vi "axis to can.vi"(5 "send speed over can":T1, 6 "ROS":bool, 7 "wej auto":T2 {"zadany" format="%<%H:%M:%S\n%x>T"}, 8 "wej ster":cluster{"Y axis":dbl, "X axis":dbl}, 9 "wej  ID":T5, 10 "wej wagi":T4, 11 "ROS in":cluster{dbl, dbl}) -> (0 "array of cans":T6[](array[typedef]) {"type" items=["CAN Data", "CAN Remote"]; "identifier" format="%.0x"}, 2 "wyj pred":cluster{i16, i16, i16, i16, i16, i16} {"?" scale=-32767.0..32767.0; "?" scale=-32767.0..32767.0; "?" scale=-32767.0..32767.0; "?" scale=-32767.0..32767.0; "?" scale=-32767.0..32767.0; "?" scale=-32767.0..32767.0}, 3 "wyj auto":T3, 4 "wyœlij":bool=TRUE)   [LabVIEW 2015]
uses:
  CANFrameControl.ctl
  PC/wyj auto.ctl
panel:
  in  "reset":bool
  out "Time has Elapsed":bool
  out "Elapsed Time (s)":dbl
  out "zadany czas":bool
  out "AUTO ?":bool
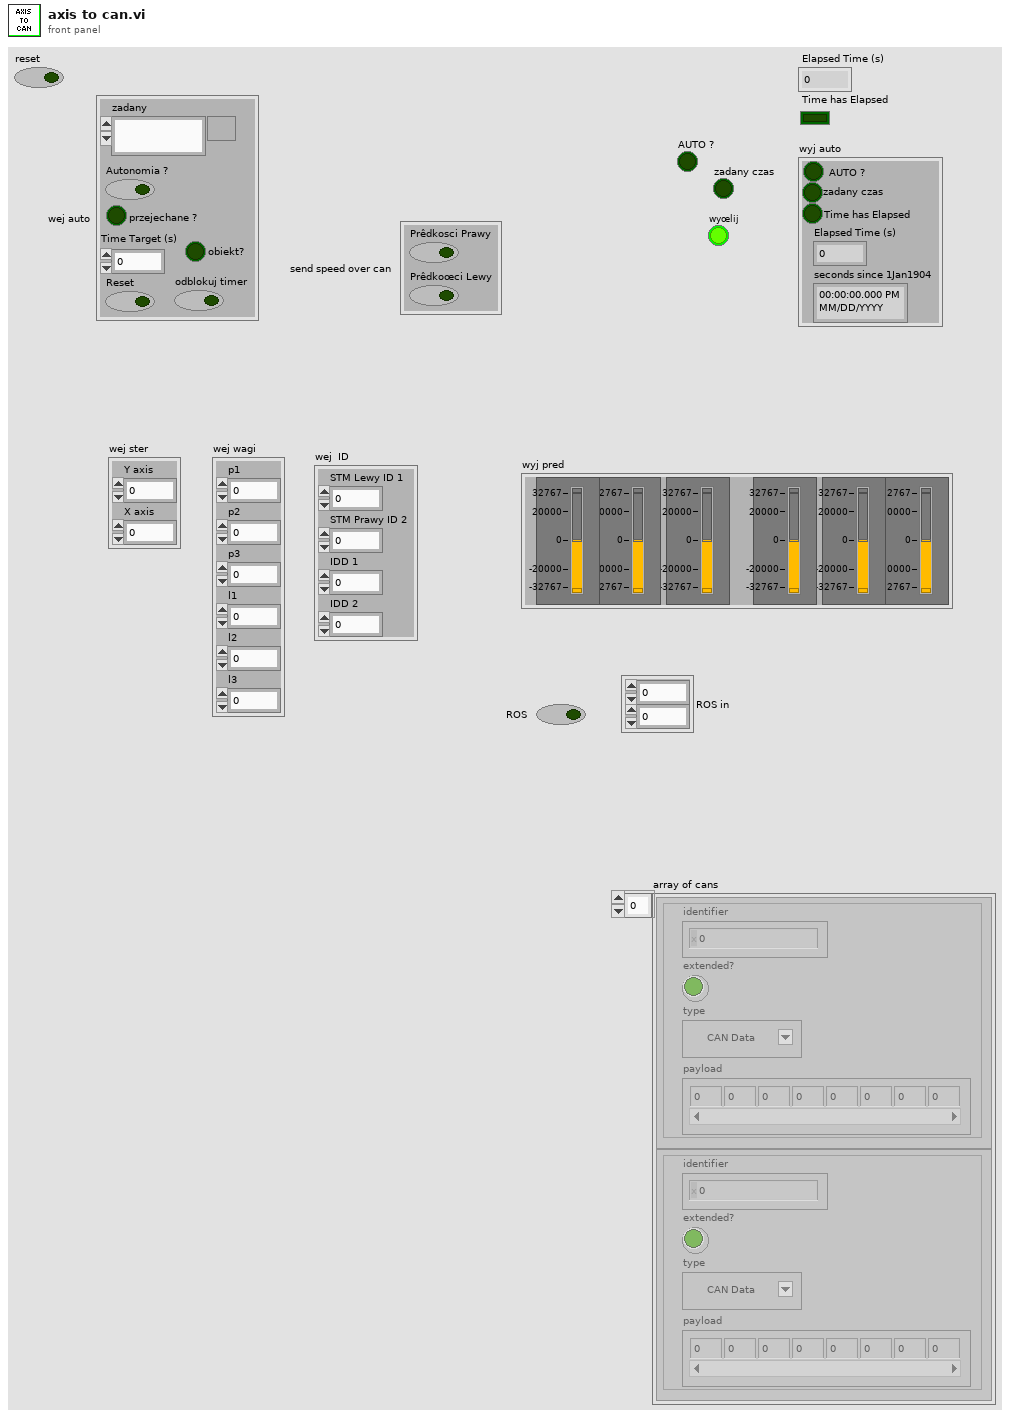
[diagram p1: front panel]
types:
  T1 = cluster{"Prêdkosci Prawy":bool, "Prêdkoœci Lewy":bool}
  T2 = cluster{"zadany":timestamp, "Autonomia ?":bool, "Time Target (s)":dbl, "Reset":bool, "odblokuj timer":bool, "obiekt?":bool, "przejechane ? ":bool}
  T3 = typedef "wyj auto.ctl" = cluster{"AUTO ?":bool, "zadany czas":bool, "Time has Elapsed":bool, "Elapsed Time (s)":dbl, "seconds since 1Jan1904":timestamp}
  T4 = cluster{"p1":dbl, "p2":dbl, "p3":dbl, "l1":dbl, "l2":dbl, "l3":dbl}
  T5 = cluster{"STM Lewy ID 1":u32, "STM Prawy ID 2":u32, "IDD 1":u8, "IDD 2":u8}
  T6 = typedef "CANFrameControl.ctl" = cluster{"identifier":u32, "extended?":bool, "type":u8, "payload":u8[]}
  T7 = cluster{bool, bool, "Time has Elapsed":bool, "Elapsed Time (s)":dbl, "seconds since 1Jan1904":timestamp}
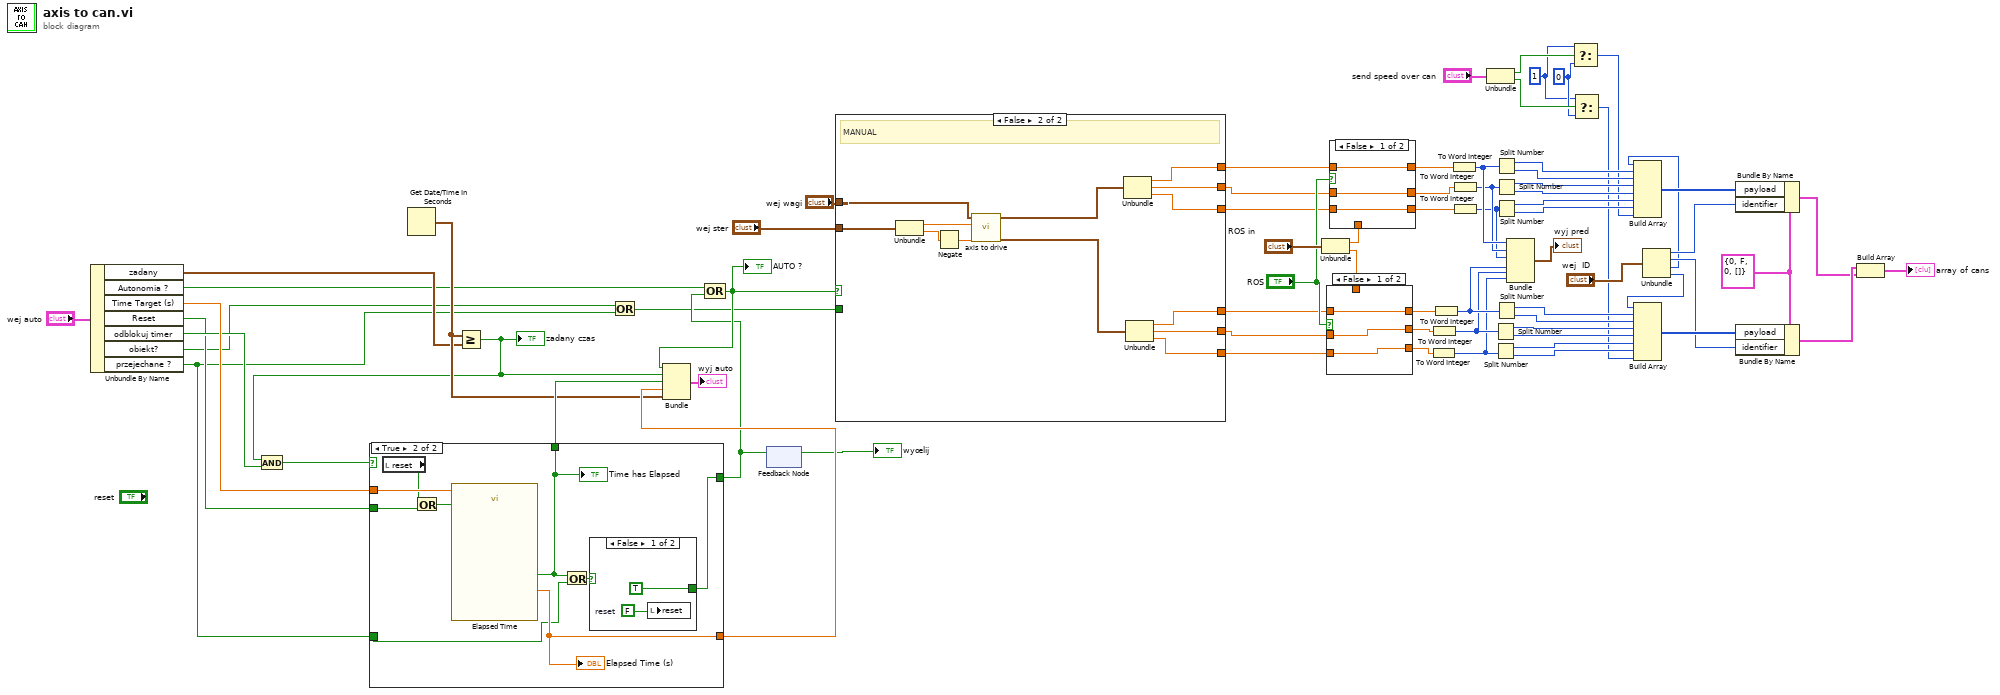
[diagram p0: block diagram]
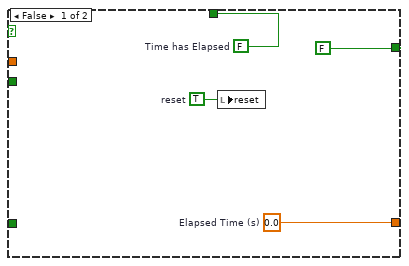
[diagram p4: hidden frame]
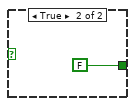
[diagram p5: hidden frame]
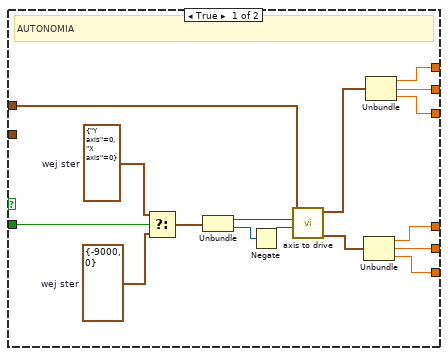
[diagram p6: hidden frame]
diagram:
  w17 = u8 1 ("element")
  w18 = u8 0 ("element")
  w72 = T6 {"identifier"=0, "extended?"=FALSE, "type"=0, "payload"=[]} ("CAN frame 2")
  n1 = Unbundle By Name("wej auto") -> ("zadany"=w36:timestamp, "Autonomia ?"=w31:bool, "Time Target (s)"=w38:dbl, "Reset"=w29:bool, "odblokuj timer"=w33:bool, "obiekt?"=w26:bool, "przejechane ?"=w24:bool)
  n2 = Get Date/Time In Seconds() -> (seconds since 1Jan1904=w37:timestamp)
  n3 = Greater Or Equal?(x=w37, y=w36) -> (x >= y?=w34:bool)
  "zadany czas" <- w34
  n4 = And(x=w34, y=w33) -> (x .and. y?=w35:bool)
  n5 = case shown="True" w35 {
    tunnel: [FALSE w86] -> w30
    tunnel: [w75 w80] -> w41
    tunnel: [w76 w79] -> w40
    tunnel: w29 -> [_ w83]
    tunnel: w38 -> [_ w85]
    tunnel: w24 -> [_ w78]
    frame False {
      w74 = TRUE  # reset
      w76 = 0.0  # Elapsed Time (s)
      w75 = FALSE  # Time has Elapsed
      n6 = local write "reset"(w74) -> ()
    }
    frame True {
      n7 = local read "reset"() -> (w82:bool)
      n8 = Or(x=w82, y=w83) -> (x .or. y?=w84:bool)
      n9 = call "Elapsed Time"("Time Target (s)"=w85, "Reset"=w84) -> ("Elapsed Time (s)"=w79:dbl, "Time has Elapsed"=w80:bool)  [unwired: 10 in, 6 out]
      "Elapsed Time (s)" <- w79
      "Time has Elapsed" <- w80
      n10 = Or(x=w80, y=w78) -> (x .or. y?=w81:bool)
      n11 = case shown="False" w81 {
        tunnel: [TRUE FALSE] -> w86
        frame False {
          w87 = FALSE  # reset
          n12 = local write "reset"(w87) -> ()
        }
        frame True {
        }
      }
    }
  }
  n13 = Or(x=w26, y=w24) -> (x .or. y?=w25:bool)
  n14 = Compound Arithmetic op=OR(w31, w30) -> (w32:bool)
  "AUTO ?" <- w32
  n15 = Bundle(w32, w34, "Time has Elapsed"=w41, "Elapsed Time (s)"=w40, "seconds since 1Jan1904"=w37) -> (→"wyj auto":T7)  [unwired: 1 in]
  n16 = feedback-in #1(w30) -> ()
  n17 = feedback #1() -> (→"wyœlij":bool)  [unwired: 1 in]
  n18 = case shown="False" w32 {
    tunnel: [w94 w107] -> w7
    tunnel: [w93 w108] -> w5
    tunnel: [w92 w106] -> w3
    tunnel: [w95 w110] -> w9
    tunnel: [w96 w111] -> w12
    tunnel: [w97 w112] -> w14
    tunnel: "wej ster" -> [_ w117]
    tunnel: "wej wagi" -> [w102 w116]
    tunnel: w25 -> [w90 _]
    frame True {
      w100 = cluster{"Y axis":i32, "X axis":i32} {"Y axis"=0, "X axis"=0}  # wej ster
      w99 = cluster{"Y axis":i32, "X axis":i32} {"Y axis"=-9000, "X axis"=0}  # wej ster
      # "AUTONOMIA"
      n19 = Select(t=w100, s=w90, f=w99) -> (s? t:f=w101:cluster{"Y axis":i32, "X axis":i32})
      n20 = Unbundle(w101) -> ("Y axis"=w103:i32, "X axis"=w105:i32)
      n21 = Negate(x=w105) -> (-x=w104:i32)
      n22 = call "axis to drive.vi"("X axis"=w104, "Y axis"=w103, "wej wagi"=w102) -> ("wyj P"=w91:cluster{"y":dbl, "y":dbl, "y":dbl}, "wyj L"=w98:cluster{"y":dbl, "y":dbl, "y":dbl})  [unwired: 7 in]
      n23 = Unbundle(w91) -> ("y"=w94:dbl, "y"=w93:dbl, "y"=w92:dbl)
      n24 = Unbundle(w98) -> ("y"=w97:dbl, "y"=w96:dbl, "y"=w95:dbl)
    }
    frame False {
      # "MANUAL"
      n25 = Unbundle(w117) -> ("Y axis"=w115:dbl, "X axis"=w118:dbl)
      n26 = Negate(x=w118) -> (-x=w114:dbl)
      n27 = call "axis to drive.vi"("X axis"=w114, "Y axis"=w115, "wej wagi"=w116) -> ("wyj P"=w109:cluster{"y":dbl, "y":dbl, "y":dbl}, "wyj L"=w113:cluster{"y":dbl, "y":dbl, "y":dbl})  [unwired: 7 in]
      n28 = Unbundle(w113) -> ("y"=w112:dbl, "y"=w111:dbl, "y"=w110:dbl)
      n29 = Unbundle(w109) -> ("y"=w107:dbl, "y"=w108:dbl, "y"=w106:dbl)
    }
  }
  n30 = Unbundle("ROS in") -> (w2:dbl, w1:dbl)
  n31 = case shown="False" "ROS" {
    tunnel: [w121 w122] -> w8
    tunnel: w7 -> [w121 _]
    tunnel: [w120 w122] -> w6
    tunnel: w5 -> [w120 _]
    tunnel: [w119 w122] -> w4
    tunnel: w3 -> [w119 _]
    tunnel: w1 -> [_ w122]
    frame False {
    }
    frame True {
    }
  }
  n32 = case shown="False" "ROS" {
    tunnel: w14 -> [w124 _]
    tunnel: [w125 w126] -> w13
    tunnel: w12 -> [w125 _]
    tunnel: [w124 w126] -> w11
    tunnel: [w123 w126] -> w10
    tunnel: w9 -> [w123 _]
    tunnel: w2 -> [_ w126]
    frame False {
    }
    frame True {
    }
  }
  n33 = To Word Integer(number=w4) -> (16bit integer=w45:i16)
  n34 = To Word Integer(number=w6) -> (16bit integer=w46:i16)
  n35 = To Word Integer(number=w8) -> (16bit integer=w47:i16)
  n36 = To Word Integer(number=w11) -> (16bit integer=w50:i16)
  n37 = To Word Integer(number=w13) -> (16bit integer=w49:i16)
  n38 = To Word Integer(number=w10) -> (16bit integer=w48:i16)
  n39 = Unbundle("send speed over can") -> ("Prêdkosci Prawy"=w22:bool, "Prêdkoœci Lewy"=w21:bool)
  n40 = Split Number(x=w46) -> (hi(x)=w59:u8, lo(x)=w58:u8)
  n41 = Split Number(x=w45) -> (hi(x)=w57:u8, lo(x)=w56:u8)
  n42 = Split Number(x=w50) -> (hi(x)=w67:u8, lo(x)=w66:u8)
  n43 = Split Number(x=w49) -> (hi(x)=w63:u8, lo(x)=w62:u8)
  n44 = Split Number(x=w48) -> (hi(x)=w61:u8, lo(x)=w60:u8)
  n45 = Split Number(x=w47) -> (hi(x)=w65:u8, lo(x)=w64:u8)
  n46 = Bundle(w50, w49, w48, w47, w46, w45) -> (→"wyj pred":cluster{i16, i16, i16, i16, i16, i16})  [unwired: 1 in]
  n47 = Select(t=w17, s=w22, f=w18) -> (s? t:f=w20:u8)
  n48 = Select(t=w17, s=w21, f=w18) -> (s? t:f=w19:u8)
  n49 = Unbundle("wej  ID") -> ("STM Lewy ID 1"=w54:u32, "STM Prawy ID 2"=w53:u32, "IDD 1"=w52:u8, "IDD 2"=w51:u8)
  n50 = Build Array(w52, w67, w66, w63, w62, w61, w60, w20) -> (w71:u8[])
  n51 = Build Array(w51, w65, w64, w59, w58, w57, w56, w19) -> (w73:u8[])
  n52 = Bundle By Name(cluster=w72, "payload"=w71, "identifier"=w54) -> (w69:T6)
  n53 = Bundle By Name(cluster=w72, "payload"=w73, "identifier"=w53) -> (w70:T6)
  n54 = Build Array(w70, w69) -> (→"array of cans":T6[])
